vi "createname.vi"(1 "Title":string, 2 "router channel":u8, 3 "threshold":cluster{"max":u32, "min":u32}) -> (0 "Title 2":string)   [LabVIEW 2009]
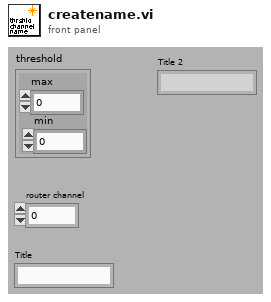
[diagram p1: front panel]
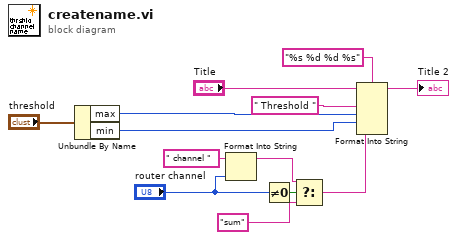
[diagram p0: block diagram]
diagram:
  n1 = Unbundle By Name("threshold") -> ("max"=w3:u32, "min"=w1:u32)
  n2 = Format Into String(initial string=" channel ", "router channel") -> (resulting string=w6:string)  [unwired: 2 in, 1 out]
  n3 = Not Equal To 0?(x="router channel") -> (x != 0?=w13:bool)
  n4 = Select(t=w6, s=w13, f="sum" ("initial string")) -> (s? t:f=w2:string)
  n5 = Format Into String(format string="%s %d %d %s", initial string="Title", " Threshold " ("input 1"), w3, w1, w2) -> (resulting string=→"Title 2":string)  [unwired: 1 in, 1 out]
